vi "Convert CFA from U32.vi"(2 "CFA in":u32 format="%x") -> (16 "CFA":T1 {"CFA" items=["CFA_NONE", "CFA_VRI", "CFA_VRIV6", "CFA_BAYER", "CFA_BAYERFLIP"]})   [LabVIEW 2013, in "VRI.lvlib"]
uses:
  VRI.lvlib
  _Type Defs/PhInt CFA.ctl
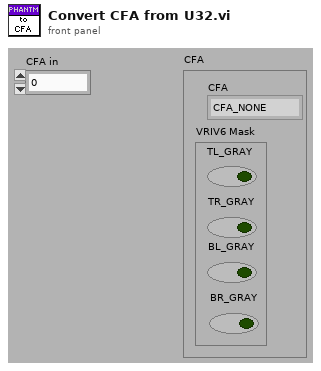
[diagram p1: front panel]
types:
  T1 = typedef "VRI.lvlib/PhInt CFA.ctl" = cluster{"CFA":u32, "VRIV6 Mask":cluster{"TL_GRAY":bool, "TR_GRAY":bool, "BL_GRAY":bool, "BR_GRAY":bool}}
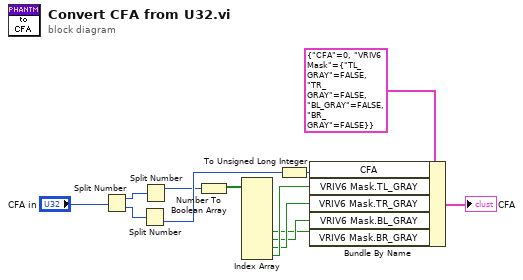
[diagram p0: block diagram]
diagram:
  n1 = Split Number(x="CFA in") -> (hi(x)=w12:u16, lo(x)=w11:u16)
  n2 = Split Number(x=w11) -> (lo(x)=w7:u8)  [unwired: 1 out]
  n3 = Split Number(x=w12) -> (hi(x)=w6:u8)  [unwired: 1 out]
  n4 = Number To Boolean Array(number=w6) -> (Boolean array=w5:bool[])
  n5 = Index Array(array=w5) -> (element #5=w1:bool, element #6=w2:bool, element #7=w3:bool, element #8=w4:bool)  [unwired: 8 in, 4 out]
  n6 = To Unsigned Long Integer(number=w7) -> (unsigned 32bit integer=w8:u32)
  n7 = Bundle By Name(cluster=T1 {"CFA"=0, "VRIV6 Mask"={"TL_GRAY"=FALSE, "TR_GRAY"=FALSE, "BL_GRAY"=FALSE, "BR_GRAY"=FALSE}} ("CFA 2"), "CFA"=w8, "VRIV6 Mask.TL_GRAY"=w4, "VRIV6 Mask.TR_GRAY"=w3, "VRIV6 Mask.BL_GRAY"=w2, "VRIV6 Mask.BR_GRAY"=w1) -> (→"CFA":T1)
